vi "subConvertCluster.vi"(1 "Input dF":dbl, 2 "Array in":cdb[](array[numeric])) -> (0 "data":cluster{"t0":dbl, "dt":dbl, "Y":cdb[]} {"Y" format="%.3f"; "dt" format="%^.2e"; "t0" format="%.4f"})   [LabVIEW 2013]
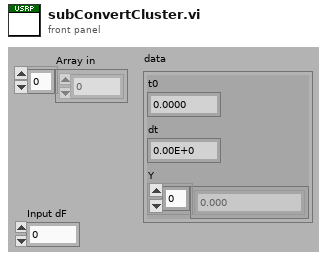
[diagram p1: front panel]
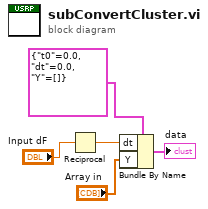
[diagram p0: block diagram]
diagram:
  n1 = Reciprocal(x="Input dF") -> (1/x=w4:dbl)
  n2 = Bundle By Name(cluster=cluster{"t0":dbl, "dt":dbl, "Y":cdb[]} {"t0"=0.0, "dt"=0.0, "Y"=[]} ("data"), "dt"=w4, "Y"="Array in") -> (→"data":cluster{"t0":dbl, "dt":dbl, "Y":cdb[]})
